vi "WaterControl.vi"() -> ()   [LabVIEW 2015]
panel:
  in  "stop":bool
  out "Estado":string="Sistema Apagado"
  out "Termometro":dbl(slide) scale=0.0..80.0
  out "Tanque":dbl(slide) scale=0.0..10.0
  out "Valvula de\nSalida":bool
  out "Calefactor":bool
  out "Bomba":bool
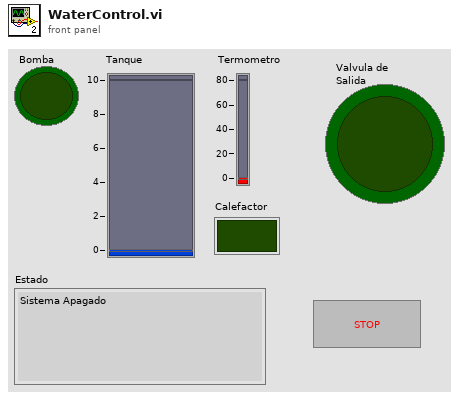
[diagram p1: front panel]
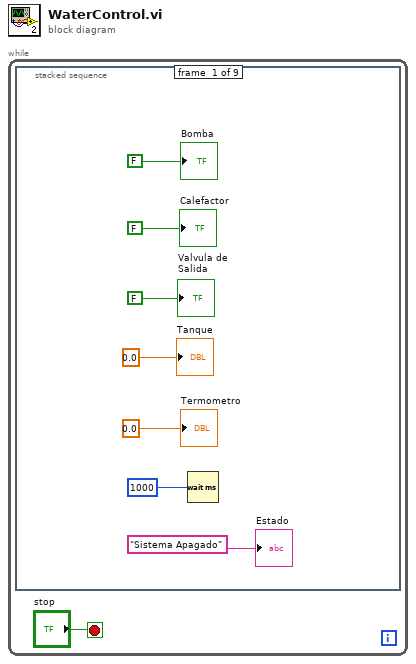
[diagram p0: block diagram]
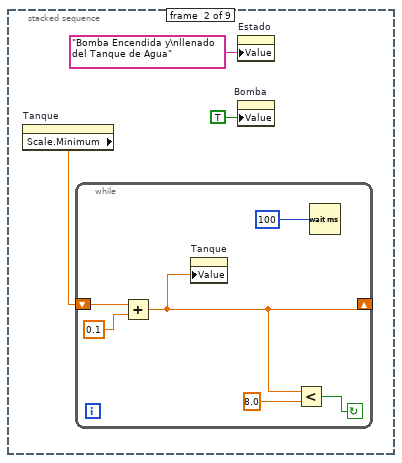
[diagram p2: hidden frame]
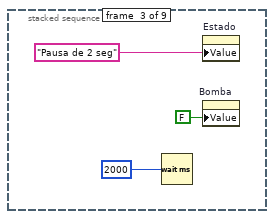
[diagram p3: hidden frame]
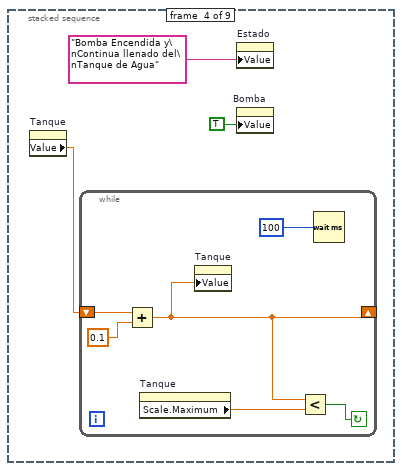
[diagram p4: hidden frame]
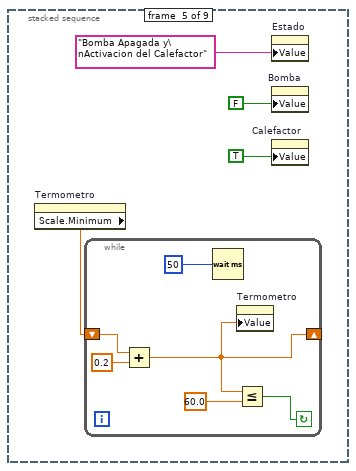
[diagram p5: hidden frame]
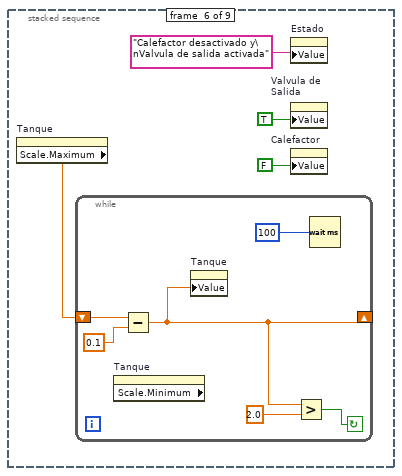
[diagram p6: hidden frame]
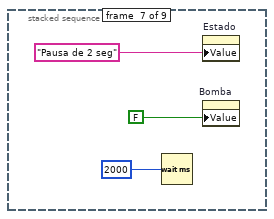
[diagram p7: hidden frame]
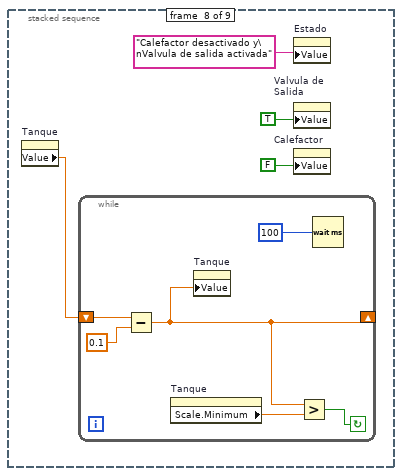
[diagram p8: hidden frame]
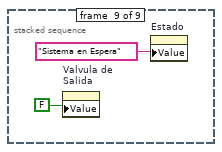
[diagram p9: hidden frame]
diagram:
  n1 = while {
    stop <- "stop" stop-if-true
    n2 = stacked-sequence {
      frame #0 {
        n3 = Wait (ms)(milliseconds to wait=u32 1000) -> ()  [unwired: 1 out]
        "Bomba" <- FALSE ("Bomba")
        "Calefactor" <- FALSE ("Calefactor")
        "Valvula de\nSalida" <- FALSE ("Valvual de Salida")
        "Tanque" <- 0.0 ("Tanque 1")
        "Termometro" <- 0.0 ("Termometro")
        "Estado" <- "Sistema Apagado"
      }
      frame #1 {
        n4 = property on="Tanque" class="Slide (strict)"() -> ("Scale.Minimum"=w9:dbl)  [unwired: 2 in, 2 out]
        n5 = while {
          shift-right: [w15] -> _
          shift-left: w9 -> [w16]
          stop <- w14 continue-if-true
          n6 = Add(x=w16, y=0.1) -> (x+y=w15:dbl)
          n7 = property on="Tanque" class="Slide (strict)"("Value"=w15) -> ()  [unwired: 2 in, 2 out]
          n8 = Less?(x=w15, y=8.0) -> (x < y?=w14:bool)
          n9 = Wait (ms)(milliseconds to wait=u32 100) -> ()  [unwired: 1 out]
        }
        n10 = property on="Estado" class="Str"("Value"="Bomba Encendida y\nllenado del Tanque de Agua") -> ()  [unwired: 2 in, 2 out]
        n11 = property on="Bomba" class="Bool (strict)"("Value"=TRUE ("Bomba")) -> ()  [unwired: 2 in, 2 out]
      }
      frame #2 {
        n12 = Wait (ms)(milliseconds to wait=u32 2000) -> ()  [unwired: 1 out]
        n13 = property on="Estado" class="Str"("Value"="Pausa de 2 seg") -> ()  [unwired: 2 in, 2 out]
        n14 = property on="Bomba" class="Bool (strict)"("Value"=FALSE ("Bomba")) -> ()  [unwired: 2 in, 2 out]
      }
      frame #3 {
        n15 = property on="Tanque" class="Slide (strict)"() -> ("Value"=w21:dbl)  [unwired: 2 in, 2 out]
        n16 = while {
          shift-right: [w27] -> _
          shift-left: w21 -> [w28]
          stop <- w26 continue-if-true
          n17 = Add(x=w28, y=0.1) -> (x+y=w27:dbl)
          n18 = property on="Tanque" class="Slide (strict)"() -> ("Scale.Maximum"=w24:dbl)  [unwired: 2 in, 2 out]
          n19 = property on="Tanque" class="Slide (strict)"("Value"=w27) -> ()  [unwired: 2 in, 2 out]
          n20 = Less?(x=w27, y=w24) -> (x < y?=w26:bool)
          n21 = Wait (ms)(milliseconds to wait=u32 100) -> ()  [unwired: 1 out]
        }
        n22 = property on="Estado" class="Str"("Value"="Bomba Encendida y\nContinua llenado del\nTanque de Agua") -> ()  [unwired: 2 in, 2 out]
        n23 = property on="Bomba" class="Bool (strict)"("Value"=TRUE ("Bomba")) -> ()  [unwired: 2 in, 2 out]
      }
      frame #4 {
        n24 = property on="Termometro" class="Slide (strict)"() -> ("Scale.Minimum"=w30:dbl)  [unwired: 2 in, 2 out]
        n25 = while {
          shift-right: [w34] -> _
          shift-left: w30 -> [w38]
          stop <- w36 continue-if-true
          n26 = Add(x=w38, y=0.2) -> (x+y=w34:dbl)
          n27 = Wait (ms)(milliseconds to wait=u32 50) -> ()  [unwired: 1 out]
          n28 = property on="Termometro" class="Slide (strict)"("Value"=w34) -> ()  [unwired: 2 in, 2 out]
          n29 = Less Or Equal?(x=w34, y=60.0) -> (x <= y?=w36:bool)
        }
        n30 = property on="Estado" class="Str"("Value"="Bomba Apagada y\nActivacion del Calefactor") -> ()  [unwired: 2 in, 2 out]
        n31 = property on="Bomba" class="Bool (strict)"("Value"=FALSE ("Bomba")) -> ()  [unwired: 2 in, 2 out]
        n32 = property on="Calefactor" class="Bool (strict)"("Value"=TRUE ("Calefactor")) -> ()  [unwired: 2 in, 2 out]
      }
      frame #5 {
        n33 = property on="Tanque" class="Slide (strict)"() -> ("Scale.Maximum"=w41:dbl)  [unwired: 2 in, 2 out]
        n34 = while {
          shift-right: [w47] -> _
          shift-left: w41 -> [w48]
          stop <- w46 continue-if-true
          n35 = property on="Tanque" class="Slide (strict)" props=["Scale", "Minimum"]() -> ()  [unwired: 2 in, 3 out]
          n36 = Subtract(x=w48, y=0.1) -> (x-y=w47:dbl)
          n37 = property on="Tanque" class="Slide (strict)"("Value"=w47) -> ()  [unwired: 2 in, 2 out]
          n38 = Greater?(x=w47, y=2.0) -> (0:w46:bool)
          n39 = Wait (ms)(milliseconds to wait=u32 100) -> ()  [unwired: 1 out]
        }
        n40 = property on="Estado" class="Str"("Value"="Calefactor desactivado y\nValvula de salida activada") -> ()  [unwired: 2 in, 2 out]
        n41 = property on="Valvula de\nSalida" class="Bool (strict)"("Value"=TRUE ("Calefactor")) -> ()  [unwired: 2 in, 2 out]
        n42 = property on="Calefactor" class="Bool (strict)"("Value"=FALSE ("Calefactor")) -> ()  [unwired: 2 in, 2 out]
      }
      frame #6 {
        n43 = Wait (ms)(milliseconds to wait=u32 2000) -> ()  [unwired: 1 out]
        n44 = property on="Estado" class="Str"("Value"="Pausa de 2 seg") -> ()  [unwired: 2 in, 2 out]
        n45 = property on="Bomba" class="Bool (strict)"("Value"=FALSE ("Bomba")) -> ()  [unwired: 2 in, 2 out]
      }
      frame #7 {
        n46 = property on="Tanque" class="Slide (strict)"() -> ("Value"=w55:dbl)  [unwired: 2 in, 2 out]
        n47 = while {
          shift-right: [w60] -> _
          shift-left: w55 -> [w61]
          stop <- w59 continue-if-true
          n48 = Subtract(x=w61, y=0.1) -> (x-y=w60:dbl)
          n49 = property on="Tanque" class="Slide (strict)"() -> ("Scale.Minimum"=w57:dbl)  [unwired: 2 in, 2 out]
          n50 = property on="Tanque" class="Slide (strict)"("Value"=w60) -> ()  [unwired: 2 in, 2 out]
          n51 = Greater?(x=w60, y=w57) -> (0:w59:bool)
          n52 = Wait (ms)(milliseconds to wait=u32 100) -> ()  [unwired: 1 out]
        }
        n53 = property on="Estado" class="Str"("Value"="Calefactor desactivado y\nValvula de salida activada") -> ()  [unwired: 2 in, 2 out]
        n54 = property on="Valvula de\nSalida" class="Bool (strict)"("Value"=TRUE ("Calefactor")) -> ()  [unwired: 2 in, 2 out]
        n55 = property on="Calefactor" class="Bool (strict)"("Value"=FALSE ("Calefactor")) -> ()  [unwired: 2 in, 2 out]
      }
      frame #8 {
        n56 = property on="Valvula de\nSalida" class="Bool (strict)"("Value"=FALSE ("Calefactor")) -> ()  [unwired: 2 in, 2 out]
        n57 = property on="Estado" class="Str"("Value"="Sistema en Espera") -> ()  [unwired: 2 in, 2 out]
      }
    }
  }
